vi "test2.vi"() -> (3 "x+1":i32)   [LabVIEW 2016]
panel:
  in  "MAIN STOP":bool
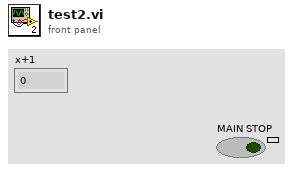
[diagram p1: front panel]
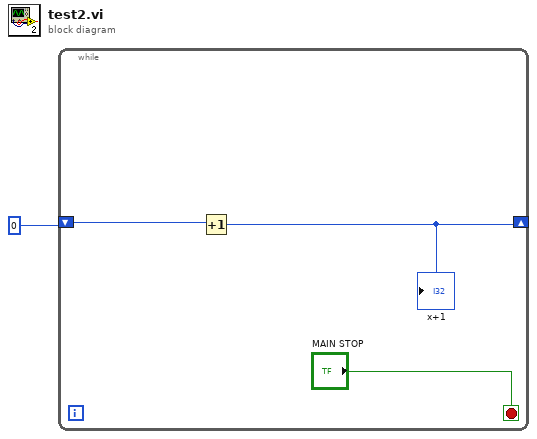
[diagram p0: block diagram]
diagram:
  n1 = while {
    shift-right: [w3] -> _
    shift-left: 0 -> [w4]
    stop <- "MAIN STOP" stop-if-true
    n2 = Increment(x=w4) -> (x+1=w3:i32)
    "x+1" <- w3
  }
